vi "BonOMM-SAOMM.vi"() -> ()   [LabVIEW 2019] (continued)
                                n2799 = Two Button Dialog(message="Voulez-vous vraiment utiliser ces \nvaleurs comme valeurs de centre (x,y)", 1:"Non" ("F button name (\"Cancel\")"), 2:"Oui" ("T button name (\"OK\")")) -> (T button?=w6859:bool)
                                n2800 = case shown="Faux" w6859 {
                                tunnel: w6858 -> [w6863 _]
                                tunnel: w6857 -> [w6864 _]
                                frame False {
                                n2801 = local write "Reference Y"(w6864) -> ()
                                n2802 = local write "Reference X"(w6863) -> ()
                                }
                                frame True {
                                }
                                }
                                }
                                }
                                }
                                }
                              }
                            }
                          }
                        }
                      }
                      frame #4 {
                        n2803 = control-ref of="PrAMS-ACK"() -> (w6876:refnum<vi>)
                        n2804 = local read "PrAMS VRN"() -> (w6899:refnum<visa-resource-name>)
                        n2805 = local read "PrAMS Error"() -> (w6898:errorcluster)
                        n2806 = local read "MessageType"() -> (w6884:cluster{string[], u32[]})
                        n2807 = control-ref of="PrAMS actif"() -> (w6877:refnum<vi>)
                        n2808 = local read "Signature"() -> (w6887:u32)
                        n2809 = call-poly "SAOMM-Num2littleEndian.vi"("Number"=w6874) -> ("LiitleEndianedData"=w6883:u8[])  [unwired: 14 in]
                        n2810 = call-poly "SAOMM-Num2littleEndian.vi"("Number"=w6873) -> ("LiitleEndianedData"=w6882:u8[])  [unwired: 14 in]
                        n2811 = call-poly "SAOMM-Num2littleEndian.vi"("Number"=w6868) -> ("LiitleEndianedData"=w6881:u8[])  [unwired: 14 in]
                        n2812 = call-poly "SAOMM-Num2littleEndian.vi"("Number"=w6867) -> ("LiitleEndianedData"=w6880:u8[])  [unwired: 14 in]
                        n2813 = call-poly "SAOMM-Num2littleEndian.vi"("Number"=w6866) -> ("LiitleEndianedData"=w6879:u8[])  [unwired: 14 in]
                        n2814 = call-poly "SAOMM-Num2littleEndian.vi"("Number"=w6865) -> ("LiitleEndianedData"=w6878:u8[])  [unwired: 14 in]
                        n2815 = call "SAOMM-SendSET.vi"("PRAMMS-COMM IN"=w6899, "Active Refnum"=w6877, "PrAMS-ACK"=w6876, "Signature"=w6887, "Error IN"=w6898, "MessageType"=w6884, "Active SET"="emtSetROIHeight", "Value (little endianed byte array)"=w6883) -> ("PRAMMS-COMM OUT"=w6897:refnum<visa-resource-name>, "Error OUT"=w6894:errorcluster)  [unwired: 4 in, 2 out]
                        n2816 = call "SAOMM-SendSET.vi"("PRAMMS-COMM IN"=w6897, "Active Refnum"=w6877, "PrAMS-ACK"=w6876, "Signature"=w6887, "Error IN"=w6894, "MessageType"=w6884, "Active SET"="emtSetROIWidth", "Value (little endianed byte array)"=w6882) -> ("PRAMMS-COMM OUT"=w6896:refnum<visa-resource-name>, "Error OUT"=w6893:errorcluster)  [unwired: 4 in, 2 out]
                        n2817 = call "SAOMM-SendSET.vi"("PRAMMS-COMM IN"=w6896, "Active Refnum"=w6877, "PrAMS-ACK"=w6876, "Signature"=w6887, "Error IN"=w6893, "MessageType"=w6884, "Active SET"="emtSetROIXReferencePoint", "Value (little endianed byte array)"=w6881) -> ("PRAMMS-COMM OUT"=w6895:refnum<visa-resource-name>, "Error OUT"=w6892:errorcluster)  [unwired: 4 in, 2 out]
                        n2818 = call "SAOMM-SendSET.vi"("PRAMMS-COMM IN"=w6895, "Active Refnum"=w6877, "PrAMS-ACK"=w6876, "Signature"=w6887, "Error IN"=w6892, "MessageType"=w6884, "Active SET"="emtSetROIYReferencePoint", "Value (little endianed byte array)"=w6880) -> ("PRAMMS-COMM OUT"=w6889:refnum<visa-resource-name>, "Error OUT"=w6888:errorcluster)  [unwired: 4 in, 2 out]
                        n2819 = call "SAOMM-SendSET.vi"("PRAMMS-COMM IN"=w6889, "Active Refnum"=w6877, "PrAMS-ACK"=w6876, "Signature"=w6887, "Error IN"=w6888, "MessageType"=w6884, "Active SET"="emtSetROIXOffset", "Value (little endianed byte array)"=w6879) -> ("PRAMMS-COMM OUT"=w6890:refnum<visa-resource-name>, "Error OUT"=w6891:errorcluster)  [unwired: 4 in, 2 out]
                        n2820 = call "SAOMM-SendSET.vi"("PRAMMS-COMM IN"=w6890, "Active Refnum"=w6877, "PrAMS-ACK"=w6876, "Signature"=w6887, "Error IN"=w6891, "MessageType"=w6884, "Active SET"="emtSetROIYOffset", "Value (little endianed byte array)"=w6878) -> ("Error OUT"=w6875:errorcluster)  [unwired: 4 in, 3 out]
                        n2821 = local write "PrAMS Error"(w6875) -> ()
                      }
                      frame #5 {
                        # "Pas certain que ce soit encore très utile ..."
                        n2822 = local write "Centrage_ready"(TRUE) -> ()
                        n2823 = global write "Globals.vi" "EXIT"(FALSE) -> ()
                        n2824 = local write "Indicateur d'état"("Centrage : fin de la routine" ("Indicateur d'état")) -> ()
                      }
                    }
                  }
                }
                n2825 = flat-sequence {
                  tunnel: [FALSE ("CentrageLed")] -> w6632
                  frame #0 {
                    "Centrage_ready" <- FALSE
                  }
                  frame #1 {
                    n2826 = while {
                      stop <- w6905 stop-if-true
                      n2827 = local read "CentrageLed"() -> (w6907:bool)
                      n2828 = Wait (ms)(milliseconds to wait=u32 250) -> ()  [unwired: 1 out]
                      n2829 = Not(x=w6907) -> (.not. x?=→"CentrageLed":bool)
                      n2830 = local read "Centrage_ready"() -> (w6905:bool)
                    }
                  }
                }
                n2831 = global write "Globals.vi" "EXIT"(FALSE ("Visible")) -> ()
                n2832 = local write "CentrageLed"(w6632) -> ()
              }
              event "ST+", "ST-": Value Change {
                n2833 = event-data() -> ()  [unwired: 1 in, 6 out]
                n2834 = Build Array("ST+", "ST-") -> (w6911:bool[])
                n2835 = Boolean Array To Number(Boolean array=w6911) -> (number=w6910:u32)
                n2836 = local read "MC-BonOMM VRN"() -> (w6909:refnum<visa-resource-name>)
                n2837 = case shown="2" w6910 {
                  tunnel: w6909 -> [_ w6916 w6936]
                  frame 0, Default {
                  }
                  frame 2 {
                    n2838 = call "MC-BonOMM_talker.vi"("MC-BonOMM VRN"=w6916, "Commande"="-" ("write buffer"), "Timeout (ms)"=1000, "answer=command?"=TRUE) -> ("ok ?"=w6914:bool)  [unwired: 1 in, 1 out]
                    n2839 = case shown="Vrai" w6914 {
                      tunnel: w6916 -> [w6919 w6930]
                      frame False {
                        n2840 = One Button Dialog(message="Erreur lors de la commande de déplacement", button name ("OK")="Ok ?!?") -> ()  [unwired: 1 out]
                        n2841 = call "MC-BonOMM_talker.vi"("MC-BonOMM VRN"=w6919, "Commande"="s" ("write buffer"), "Timeout (ms)"=1000, "answer=command?"=TRUE) -> ()  [unwired: 1 in, 2 out]
                      }
                      frame True {
                        n2842 = while {
                          tunnel: w6930 -> [w6932]
                          tunnel: [w6932] -> w6929
                          stop <- w6931 continue-if-true
                          n2843 = local read "ST-"() -> (w6931:bool)
                          n2844 = Wait (ms)(milliseconds to wait=u32 50) -> ()  [unwired: 1 out]
                        }
                        n2845 = call "MC-BonOMM_talker.vi"("MC-BonOMM VRN"=w6929, "Commande"="s" ("write buffer"), "Timeout (ms)"=1000, "answer=command?"=TRUE) -> ("ok ?"=w6925:bool)  [unwired: 1 in, 1 out]
                        n2846 = local write "MC_connect"(w6925) -> ()
                      }
                    }
                    n2847 = local write "MC_connect"(w6914) -> ()
                  }
                  frame 1 {
                    n2848 = call "MC-BonOMM_talker.vi"("MC-BonOMM VRN"=w6936, "Commande"="+" ("write buffer"), "Timeout (ms)"=1000, "answer=command?"=TRUE) -> ("ok ?"=w6934:bool)  [unwired: 1 in, 1 out]
                    n2849 = case shown="Vrai" w6934 {
                      tunnel: w6936 -> [w6940 w6951]
                      frame False {
                        n2850 = One Button Dialog(message="Erreur lors de la commande de déplacement", button name ("OK")="Ok ?!?") -> ()  [unwired: 1 out]
                        n2851 = call "MC-BonOMM_talker.vi"("MC-BonOMM VRN"=w6940, "Commande"="s" ("write buffer"), "Timeout (ms)"=1000, "answer=command?"=TRUE) -> ("ok ?"=w6939:bool)  [unwired: 1 in, 1 out]
                        n2852 = local write "MC_connect"(w6939) -> ()
                      }
                      frame True {
                        n2853 = while {
                          tunnel: w6951 -> [w6953]
                          tunnel: [w6953] -> w6950
                          stop <- w6952 continue-if-true
                          n2854 = local read "ST+"() -> (w6952:bool)
                          n2855 = Wait (ms)(milliseconds to wait=u32 50) -> ()  [unwired: 1 out]
                        }
                        n2856 = call "MC-BonOMM_talker.vi"("MC-BonOMM VRN"=w6950, "Commande"="s" ("write buffer"), "Timeout (ms)"=1000, "answer=command?"=TRUE) -> ("ok ?"=w6946:bool)  [unwired: 1 in, 1 out]
                        n2857 = local write "MC_connect"(w6946) -> ()
                      }
                    }
                    n2858 = local write "MC_connect"(w6934) -> ()
                  }
                }
              }
              event "Ajust z to tel": Value Change {
                n2859 = event-data() -> ()  [unwired: 1 in, 6 out]
                n2860 = local read "Foyer"() -> (w6955:dbl)
                n2861 = case shown="Vrai" "Ajust z to tel" {
                  tunnel: w6955 -> [_ w6971]
                  frame False {
                  }
                  frame True {
                    n2862 = local read "k0_focus"() -> (w6967:dbl)
                    n2863 = local read "k1_focus"() -> (w6966:dbl)
                    n2864 = formula code="foyersonde=foyertel*k1+k0;"("foyertel"=w6971, "k0"=w6967, "k1"=w6966) -> ("foyersonde"=w6958:dbl)
                    n2865 = local read "CentreTel X"() -> (w6965:dbl)
                    n2866 = local read "CentreTel Y"() -> (w6964:dbl)
                    n2867 = local read "Position X"() -> (w6960:dbl)
                    n2868 = local read "Position Y"() -> (w6959:dbl)
                    n2869 = local read "a1_focus"() -> (w6963:dbl)
                    n2870 = local read "a2_focus"() -> (w6962:dbl)
                    n2871 = local read "a3_focus"() -> (w6961:dbl)
                    n2872 = control-ref of="TERMINAL"() -> (w6969:refnum<vi>)
                    n2873 = control-ref of="Indicateur d'état"() -> (w6970:refnum<vi>)
                    n2874 = call "Calc_focus.vi"("Pos X"=w6960, "a0"=w6958, "Pos Y"=w6959, "Cen X"=w6965, "Cen Y"=w6964, "a1"=w6963, "a2"=w6962, "a3"=w6961) -> ("Foyer"=w6957:dbl)  [unwired: 6 in, 1 out]
                    n2875 = call "TERMINAL.vi"("Indicateur Refnum"=w6970, "Terminal Refnum"=w6969, "Indicateur d'état"="Ajustement automatique du foyer de la caméra de guidage") -> ()
                    n2876 = local write "FoyerAuCentre"(w6958) -> ()
                    n2877 = property on="FoyerTable" class="NumNb (strict)"("Val(Sgnl)"=w6957) -> ()  [unwired: 2 in, 2 out]
                  }
                }
              }
              event "Foyer+", "Foyer-": Mouse Down {
                n2878 = event-data() -> ()  [unwired: 1 in, 8 out]
                n2879 = Or(x="Foyer+", y="Foyer-") -> (x .or. y?=w6973:bool)
                n2880 = case shown="Vrai" w6973 {
                  tunnel: "Foyer+" -> [_ w6997]
                  frame False {
                  }
                  frame True {
                    w6983 = "AZ" ("StageTag")
                    n2881 = local read "vitesse focus"() -> (w6996:dbl)
                    n2882 = control-ref of="TERMINAL"() -> (w6988:refnum<vi>)
                    n2883 = control-ref of="Indicateur d'état"() -> (w6987:refnum<vi>)
                    n2884 = Negate(x=w6996) -> (-x=w6995:dbl)
                    n2885 = local write "Focusing"(TRUE ("Focusing")) -> ()
                    n2886 = Select(t=w6996, s=w6997, f=w6995) -> (s? t:f=w6982:dbl)
                    n2887 = local read "Table VRN"() -> (w6994:refnum<visa-resource-name>)
                    n2888 = local read "Table Error"() -> (w6993:errorcluster)
                    n2889 = call "TERMINAL.vi"("Indicateur Refnum"=w6987, "Terminal Refnum"=w6988, "Indicateur d'état"="Modification du foyer \"au centre\" de la caméra de guidage") -> ()
                    n2890 = control-ref of="Table actif"() -> (w6990:refnum<vi>)
                    n2891 = call "Newmark-Jog.vi"("Table VRN IN"=w6994, "StageTag"=w6983, "Bool Refnum"=w6990, "Error IN"=w6993, "Velocity"=w6982) -> ("Table VRN OUT"=w6991:refnum<visa-resource-name>, "Error OUT"=w6992:errorcluster)  [unwired: 9 in]
                    n2892 = flat-sequence {
                      tunnel: w6991 -> [w7001]
                      tunnel: w6992 -> [w7000]
                      tunnel: [w7001] -> w6986
                      tunnel: [w7000] -> w6985
                      tunnel: [w6999] -> w6984
                      tunnel: w6983 -> [w6999]
                      tunnel: [w6998] -> _
                      tunnel: w6985 -> [w7013]
                      tunnel: w6986 -> [w7014]
                      tunnel: [w7011] -> w6981
                      tunnel: [w7010] -> w6979
                      tunnel: [w7012] -> w6977
                      tunnel: w6984 -> [w7012]
                      tunnel: w6981 -> [w7018]
                      tunnel: [w7018] -> w6980
                      tunnel: w6979 -> [w7017]
                      tunnel: [w7017] -> w6978
                      tunnel: w6977 -> [w7016]
                      tunnel: [w7016] -> w6976
                      tunnel: w6980 -> [w7029]
                      tunnel: w6978 -> [w7028]
                      tunnel: w6976 -> [w7027]
                      frame #0 {
                        n2893 = while {
                          tunnel: [w7002] -> w6998
                          stop <- w7004 continue-if-true
                          n2894 = local read "Exceptions"() -> (w7003:T3)
                          n2895 = local read "Foyer-"() -> (w7007:bool)
                          n2896 = local read "Foyer+"() -> (w7008:bool)
                          n2897 = Unbundle By Name(w7003) -> ("Overtravel"=w7002:bool)
                          n2898 = Or(x=w7008, y=w7007) -> (x .or. y?=w7005:bool)
                          n2899 = Wait (ms)(milliseconds to wait=u32 100) -> ()  [unwired: 1 out]
                          n2900 = Not(x=w7002) -> (.not. x?=w7006:bool)
                          n2901 = And(x=w7005, y=w7006) -> (x .and. y?=w7004:bool)
                        }
                      }
                      frame #1 {
                        n2902 = control-ref of="Table actif"() -> (w7015:refnum<vi>)
                        n2903 = call "Newmark-Stop.vi"("Table VRN IN"=w7014, "Bool Refnum"=w7015, "Error IN"=w7013) -> ("Table VRN OUT"=w7011:refnum<visa-resource-name>, "Error OUT"=w7010:errorcluster)  [unwired: 11 in]
                      }
                      frame #2 {
                        n2904 = while {
                          stop <- w7020 continue-if-true
                          n2905 = local read "MovingZ"() -> (w7020:bool)
                          n2906 = Wait (ms)(milliseconds to wait=u32 100) -> ()  [unwired: 1 out]
                        }
                      }
                      frame #3 {
                        n2907 = local read "vitesse rapide"() -> (w7024:dbl)
                        n2908 = local read "vitesse lente"() -> (w7025:dbl)
                        n2909 = local read "accelleration"() -> (w7023:dbl)
                        n2910 = control-ref of="Table actif"() -> (w7026:refnum<vi>)
                        n2911 = call "Newmark-SetSpeed.vi"("Table VRN"=w7029, "StageTAG"=w7027, "Bool Refnum"=w7026, "Error IN"=w7028, "Vitesse Lente"=w7025, "Vitesse Rapide"=w7024, "Accélération"=w7023) -> ("Table VRN OUT"=w7022:refnum<visa-resource-name>, "Error OUT"=w7021:errorcluster)  [unwired: 6 in, 1 out]
                        n2912 = local write "Table VRN"(w7022) -> ()
                        n2913 = local write "Table Error"(w7021) -> ()
                      }
                    }
                  }
                }
              }
              event "FoyerTable": Value Change {
                n2914 = event-data() -> ("NewVal"=w7032:dbl)  [unwired: 1 in, 5 out]
                n2915 = local write "Cible Z"(w7032) -> ()
                n2916 = local read "Table VRN"() -> (w7039:refnum<visa-resource-name>)
                n2917 = local read "Table Error"() -> (w7037:errorcluster)
                n2918 = control-ref of="Table actif"() -> (w7035:refnum<vi>)
                n2919 = local write "CorrectZ"(TRUE ("CorrectZ")) -> ()
                n2920 = call "Newmark-GotoOne.vi"("Table VRN IN"=w7039, "Bool Refnum"=w7035, "StageTAG"="AZ", "Notify?"=FALSE, "Error IN"=w7037, "Position"=w7032) -> ("Table VRN OUT"=w7038:refnum<visa-resource-name>, "Error OUT"=w7036:errorcluster)  [unwired: 8 in]
                n2921 = local write "Focusing"(TRUE ("Focusing")) -> ()
                n2922 = local write "Table VRN"(w7038) -> ()
                n2923 = local write "Table Error"(w7036) -> ()
                n2924 = Unbundle By Name(w7036) -> ("status"=w7040:bool)
                n2925 = Not(x=w7040) -> ()  [unwired: 1 out]
              }
              event "ApplyCorrection": Value Change {
                n2926 = event-data() -> ()  [unwired: 1 in, 6 out]
                n2927 = local read "ApplyCorrection"() -> (w7041:bool)
                n2928 = case shown="Vrai" w7041 {
                  frame False {
                  }
                  frame True {
                    n2929 = local read "Cible X"() -> (w7047:dbl)
                    n2930 = local read "Position X"() -> (w7044:dbl)
                    n2931 = local read "Cible Y"() -> (w7045:dbl)
                    n2932 = local read "Position Y"() -> (w7046:dbl)
                    n2933 = local read "Cible Z"() -> (w7049:dbl)
                    n2934 = local read "Position Z"() -> (w7048:dbl)
                    n2935 = Subtract(x=w7045, y=w7046) -> (x-y=w7042:dbl)
                    n2936 = Subtract(x=w7047, y=w7044) -> (x-y=w7043:dbl)
                    n2937 = Subtract(x=w7049, y=w7048) -> (x-y=w7053:dbl)
                    n2938 = local read "Table Error"() -> (w7057:errorcluster)
                    n2939 = local read "Table VRN"() -> (w7058:refnum<visa-resource-name>)
                    n2940 = Build Array(w7043, w7042, w7053) -> (w7052:dbl[])
                    n2941 = control-ref of="Table actif"() -> (w7056:refnum<vi>)
                    n2942 = local write "ApplyCorrection"(FALSE ("Correct")) -> ()
                    n2943 = call "Newmark-CorrectPosition.vi"("Table VRN IN"=w7058, "Bool Refnum"=w7056, "Error IN"=w7057, "StageTags"=string[] ["AX", "AY", "AZ"], "Corrections"=w7052) -> ("Table VRN OUT"=w7055:refnum<visa-resource-name>, "Error OUT"=w7054:errorcluster)  [unwired: 8 in, 1 out]
                    n2944 = local write "Table VRN"(w7055) -> ()
                    n2945 = local write "Table Error"(w7054) -> ()
                  }
                }
              }
              event "YReference", "XReference": Value Change {
                n2946 = event-data() -> ()  [unwired: 1 in, 6 out]
                n2947 = control-ref of="ImgArray"() -> (w7067:refnum<vi>)
                n2948 = local read "ROIHeight"() -> (w7065:u16)
                n2949 = local read "ROIWidth"() -> (w7066:u16)
                n2950 = call "SAOMM-Cursor2ROI.vi"("ImgRef"=w7067, "CursorX"="XReference", "CursorY"="YReference", "ROIWidth"=w7066, "ROIHeight"=w7065) -> ("ROIXOffset"=w7064:u16, "ROIYOffset"=w7063:u16)  [unwired: 7 in, 2 out]
                n2951 = flat-sequence {
                  tunnel: w7064 -> [w7069]
                  tunnel: w7063 -> [w7068]
                  tunnel: [w7069] -> w7060
                  tunnel: [w7068] -> w7059
                  tunnel: w7060 -> [w7075]
                  tunnel: w7059 -> [w7074]
                  frame #0 {
                    n2952 = local write "ROIXOffset"(w7069) -> ()
                    n2953 = local write "ROIYOffset"(w7068) -> ()
                  }
                  frame #1 {
                    n2954 = local read "Binning"() -> (w7095:u16)
                    n2955 = local read "ROIWidth"() -> (w7089:u16)
                    n2956 = local read "ROIHeight"() -> (w7090:u16)
                    n2957 = local read "Naxis1"() -> (w7093:u16)
                    n2958 = local read "Naxis2"() -> (w7092:u16)
                    n2959 = local read "XROIRef"() -> (w7087:dbl)
                    n2960 = local read "YROIRef"() -> (w7073:dbl)
                    n2961 = Bundle("ROIXOffset"=w7075, "ROIYOffset"=w7074) -> (w7091:cluster{"ROIXOffset":u16, "ROIYOffset":u16})  [unwired: 1 in]
                    n2962 = Bundle("Naxis1"=w7093, "Naxis2"=w7092) -> (w7094:cluster{"Naxis1":u16, "Naxis2":u16})  [unwired: 1 in]
                    n2963 = Bundle("ROIWidth"=w7089, "ROIHeight"=w7090) -> (w7070:cluster{"ROIWidth":u16, "ROIHeight":u16})  [unwired: 1 in]
                    n2964 = Bundle("XROIRef"=w7087, "YROIRef"=w7073) -> (w7088:cluster{"XROIRef":dbl, "YROIRef":dbl})  [unwired: 1 in]
                    n2965 = call "SAOMM-ROI_Fixer.vi"("Binning"=w7095, "Use Offset?"=TRUE, "naxis"=w7094, "ROI"=w7070, "Offset"=w7091, "Reference Pixel"=w7088) -> ("FixedOffset"=w7078:cluster{"ROIXOffset":u16, "ROIYOffset":u16}, "FixedPixel"=w7076:cluster{"PixelX":dbl, "PixelY":dbl})  [unwired: 6 in, 2 out]
                    n2966 = Unbundle By Name(w7078) -> ("ROIXOffset"=w7086:u16, "ROIYOffset"=w7085:u16)
                    n2967 = control-ref of="PrAMS-ACK"() -> (w7098:refnum<vi>)
                    n2968 = local read "MessageType"() -> (w7097:cluster{string[], u32[]})
                    n2969 = control-ref of="PrAMS actif"() -> (w7103:refnum<vi>)
                    n2970 = local read "PrAMS VRN"() -> (w7102:refnum<visa-resource-name>)
                    n2971 = local read "PrAMS Error"() -> (w7101:errorcluster)
                    n2972 = Unbundle By Name(w7076) -> ("PixelX"=w7079:dbl, "PixelY"=w7082:dbl)
                    n2973 = To Double Precision Float(number=w7086) -> (double precision float=w7081:dbl)
                    n2974 = To Double Precision Float(number=w7085) -> (double precision float=w7080:dbl)
                    n2975 = Bundle("ROIYOffset"=w7085, "ROIXOffset"=w7086) -> (w7077:cluster{"ROIYOffset":u16, "ROIXOffset":u16})  [unwired: 1 in]
                    n2976 = Add(x=w7080, y=w7079) -> (x+y=w7072:dbl)
                    n2977 = Add(x=w7081, y=w7082) -> (x+y=w7071:dbl)
                    n2978 = call "SAOMM-UpdateROI.vi"("PRAMMS-COMM IN"=w7102, "Active Refnum"=w7103, "PrAMS-ACK"=w7098, "MessageType"=w7097, "Error IN"=w7101, "Position"=w7077) -> ("PRAMMS-COMM OUT"=w7100:refnum<visa-resource-name>, "Error OUT"=w7099:errorcluster)  [unwired: 7 in, 1 out]
                    n2979 = property on="ImgArray" class="GraphInt (strict)"() -> ("Cursor.Cursor Position"=w7084:T45)  [unwired: 2 in, 2 out]
                    n2980 = local write "XReference"(w7072) -> ()
                    n2981 = local write "YReference"(w7071) -> ()
                    n2982 = local write "PrAMS Error"(w7099) -> ()
                    n2983 = local write "PrAMS VRN"(w7100) -> ()
                    n2984 = Bundle(cluster=w7084, "Cursor X"=w7072, "Cursor Y"=w7071) -> (w7083:T45)
                    n2985 = property on="ImgArray" class="GraphInt (strict)"("Cursor.Cursor Position"=w7083) -> ()  [unwired: 2 in, 2 out]
                  }
                }
              }
              event "go Ouest", "go Nord", "go Est", "go Sud": Mouse Down {
                n2986 = event-data() -> ()  [unwired: 1 in, 8 out]
                n2987 = Compound Arithmetic op=OR("go Nord", "go Sud", "go Est", "go Ouest") -> (w7104:bool)
                n2988 = local write "enfoncé"(w7104) -> ()
                n2989 = case shown="Vrai" w7104 {
                  tunnel: "go Nord" -> [_ w7113]
                  tunnel: "go Sud" -> [_ w7112]
                  tunnel: "go Est" -> [_ w7111]
                  tunnel: "go Ouest" -> [_ w7110]
                  frame False {
                  }
                  frame True {
                    n2990 = local read "act_sonde"() -> (w7109:bool)
                    n2991 = Build Array(w7113, w7112, w7111, w7110) -> (w7115:bool[])
                    n2992 = Boolean Array To Number(Boolean array=w7115) -> (number=w7114:u32)
                    n2993 = case shown="Vrai" w7109 {
                      tunnel: w7114 -> [w7121 w7178]
                      frame False {
                        # "0.1=1'/sec"
                        n2994 = local read "FieldAstrom"() -> (w7119:T4)
                        n2995 = local read "ImgAstrom"() -> (w7118:T4)
                        n2996 = while {
                          tunnel: w7121 -> [w7139]
                          tunnel: 0.1 ("t") -> [w7136]
                          tunnel: w7119 -> [w7130]
                          tunnel: w7118 -> [w7133]
                          tunnel: [FALSE] -> w7117
                          tunnel: u32 0 ("Active Cursor") -> [w7122]
                          stop <- w7134 continue-if-true
                          n2997 = property on="TableXYPos" class="GraphXY (strict)"("Active Cursor"=w7122) -> (error out=w7126:errorcluster)  [unwired: 2 in, 1 out]
                          n2998 = property on="TableXYPos" class="GraphXY (strict)"(error in=w7126) -> (error out=w7124:errorcluster, "Cursor.Cursor Position"=w7125:T45)  [unwired: 1 in, 1 out]
                          n2999 = Unbundle(w7125) -> ("Cursor X"=w7138:dbl, "Cursor Y"=w7137:dbl)
                          n3000 = case shown="0, Par défaut" w7139 {
                            tunnel: [w7161 w7162 w7166 w7171 w7175] -> w7131
                            tunnel: w7138 -> [w7161 w7162 w7166 w7173 w7177]
                            tunnel: [w7160 w7163 w7168 w7170 w7176] -> w7132
                            tunnel: w7137 -> [w7160 w7165 w7167 w7170 w7176]
                            tunnel: w7136 -> [_ w7164 w7169 w7172 w7174]
                            frame 0, Default {
                            }
                            frame 1 {
                              n3001 = Add(x=w7165, y=w7164) -> (x+y=w7163:dbl)
                            }
                            frame 2 {
                              n3002 = Subtract(x=w7167, y=w7169) -> (x-y=w7168:dbl)
                            }
                            frame 4 {
                              n3003 = Add(x=w7173, y=w7172) -> (x+y=w7171:dbl)
                            }
                            frame 8 {
                              n3004 = Subtract(x=w7177, y=w7174) -> (x-y=w7175:dbl)
                            }
                          }
                          n3005 = Wait (ms)(milliseconds to wait=u32 100) -> ()  [unwired: 1 out]
                          n3006 = Bundle("Cursor X"=w7131, "Cursor Y"=w7132) -> (w7140:cluster{"Cursor X":dbl, "Cursor Y":dbl})  [unwired: 1 in]
                          n3007 = property on="TableXYPos" class="GraphXY (strict)"(error in=w7124, "Cursor.Cursor Position"=w7140) -> ()  [unwired: 1 in, 2 out]
                          n3008 = call "xy2ad.vi"("Y (px)"=w7132, "X (px)"=w7131, "Astrometry"=w7130) -> ("DEC (°)"=w7128:dbl, "RA (°)"=w7129:dbl)  [unwired: 5 in, 2 out]
                          n3009 = local read "ImageDSSLed"() -> (w7123:bool)
                          n3010 = case shown="Vrai" w7123 {
                            tunnel: w7133 -> [_ w7149]
                            tunnel: w7129 -> [_ w7148]
                            tunnel: w7128 -> [_ w7147]
                            frame False {
                            }
                            frame True {
                              w7145 = u16 1 items=["Region d'intérêt", "Prévisualisation", "Idle"] ("ImageUsage")
                              n3011 = call "ad2xy.vi"("DEC"=w7147, "RA"=w7148, "Astrometry"=w7149) -> ("Y"=w7151:dbl, "X"=w7152:dbl)  [unwired: 6 in, 1 out]
                              n3012 = local read "ImgData"() -> (w7157:sgl[][])
                              n3013 = To Long Integer(number=w7152) -> (32bit integer=w7155:i32)
                              n3014 = To Long Integer(number=w7151) -> (32bit integer=w7156:i32)
                              n3015 = call "subimage.vi"("Ysz/2"=100 ("Xsz/2"), "Xsz/2"=100, "Yc"=w7156, "Xc"=w7155, "ImgData"=w7157) -> ("SubImg"=w7158:sgl[][])  [unwired: 6 in]
                              n3016 = local write "SubIMG4DSS?"(TRUE ("SubIMG4DSS?")) -> ()
                              n3017 = Array Max & Min(array=w7158) -> (max value=w7159:sgl)  [unwired: 3 out]
                              n3018 = local write "ImageUsage"(w7145) -> ()
                              n3019 = call "Draw_crosshair.vi"("Image IN"=w7158, "White Value"=w7159) -> ("Image OUT"=w7150:sgl[][])  [unwired: 13 in]
                              n3020 = local write "subimg"(w7150) -> ()
                            }
                          }
                          n3021 = local read "go Nord"() -> (w7142:bool)
                          n3022 = local read "go Ouest"() -> (w7144:bool)
                          n3023 = local read "go Est"() -> (w7143:bool)
                          n3024 = local read "go Sud"() -> (w7141:bool)
                          n3025 = Compound Arithmetic op=OR(w7144, w7143, w7142, w7141) -> (w7134:bool)
                          n3026 = local write "enfoncé"(w7134) -> ()
                        }
                        n3027 = local write "go Nord"(w7117) -> ()
                        n3028 = local write "go Ouest"(w7117) -> ()
                        n3029 = local write "go Est"(w7117) -> ()
                        n3030 = local write "go Sud"(w7117) -> ()
                        n3031 = local write "enfoncé"(w7117) -> ()
                      }
                      frame True {
                        n3032 = flat-sequence {
                          tunnel: w7178 -> [w7180]
                          frame #0 {
                            # "Vrai = buggy continuous\nFaux = nouveau pas-à-pas"
                            n3033 = case shown="Faux" FALSE {
                              tunnel: w7180 -> [w7182 w7227]
                              frame False {
                                n3034 = flat-sequence {
                                tunnel: w7182 -> [w7184]
                                tunnel: [w7184] -> w7181
                                tunnel: w7181 -> [w7203]
                                frame #0 {
                                w7183 = FALSE ("go Ouest")
                                n3035 = local write "go Nord"(w7183) -> ()
                                n3036 = local write "go Ouest"(w7183) -> ()
                                n3037 = local write "go Est"(w7183) -> ()
                                n3038 = local write "go Sud"(w7183) -> ()
                                n3039 = local write "enfoncé"(w7183) -> ()
                                }
                                frame #1 {
                                # "Devrait être remplacé par la valeur théorique ..."
                                n3040 = property on="TableXYPos" class="GraphXY (strict)"("Active Cursor"=u32 1) -> (error out=w7206:errorcluster)  [unwired: 2 in, 1 out]
                                n3041 = property on="TableXYPos" class="GraphXY (strict)"(error in=w7206) -> ("Cursor.Cursor Position"=w7204:T45)  [unwired: 1 in, 2 out]
                                n3042 = Unbundle(w7204) -> ("Cursor X"=w7208:dbl, "Cursor Y"=w7207:dbl)
                                n3043 = case shown="1" w7203 {
                                tunnel: [w7210 w7211 w7215 w7220 w7224] -> w7201
                                tunnel: w7208 -> [w7210 w7211 w7215 w7222 w7226]
                                tunnel: [w7209 w7212 w7217 w7219 w7225] -> w7200
                                tunnel: w7207 -> [w7209 w7214 w7216 w7219 w7225]
                                tunnel: "ClickJOG" -> [_ w7213 w7218 w7221 w7223]
                                frame 0, Default {
                                }
                                frame 1 {
                                n3044 = Add(x=w7214, y=w7213) -> (x+y=w7212:dbl)
                                }
                                frame 2 {
                                n3045 = Subtract(x=w7216, y=w7218) -> (x-y=w7217:dbl)
                                }
                                frame 4 {
                                n3046 = Add(x=w7222, y=w7221) -> (x+y=w7220:dbl)
                                }
                                frame 8 {
                                n3047 = Subtract(x=w7226, y=w7223) -> (x-y=w7224:dbl)
                                }
                                }
                                n3048 = local read "BrasPesto"() -> (w7186:bool)
                                n3049 = local read "LimXPesto"() -> (w7185:dbl)
                                n3050 = local read "FieldAstrom"() -> (w7199:T4)
                                n3051 = call "xy2ad.vi"("Y (px)"=w7200, "X (px)"=w7201, "Astrometry"=w7199) -> ("DEC (°)"=w7197:dbl, "RA (°)"=w7198:dbl)  [unwired: 5 in, 2 out]
                                n3052 = local read "Position Z"() -> (w7193:dbl)
                                n3053 = local read "TableAstrom"() -> (w7196:T4)
                                n3054 = call "ad2xy.vi"("DEC"=w7197, "RA"=w7198, "Astrometry"=w7196) -> ("Y"=w7195:dbl, "X"=w7194:dbl)  [unwired: 6 in, 1 out]
                                n3055 = local read "Table VRN"() -> (w7191:refnum<visa-resource-name>)
                                n3056 = local read "Table Error"() -> (w7190:errorcluster)
                                n3057 = control-ref of="Table actif"() -> (w7192:refnum<vi>)
                                n3058 = call "Newmark-GotoAll.vi"("Table VRN IN"=w7191, "BrasPesto"=w7186, "Bool Refnum"=w7192, "LimXPesto"=w7185, "Notify?"=FALSE, "Error IN"=w7190, "Position X"=w7194, "Position Y"=w7195, "Position Z"=w7193) -> ("Table VRN OUT"=w7189:refnum<visa-resource-name>, "Error OUT"=w7188:errorcluster)  [unwired: 5 in]
                                n3059 = local write "Table Error"(w7188) -> ()
                                n3060 = local write "Table VRN"(w7189) -> ()
                                n3061 = local write "Cible X"(w7194) -> ()
                                n3062 = local write "Cible Z"(w7193) -> ()
                                n3063 = local write "Cible Y"(w7195) -> ()
                                }
                                }
                              }
                              frame True {
                                n3064 = stacked-sequence {
                                tunnel: w7227 -> [w7241 _]
                                frame #0 {
                                # "Est (180)"
                                # "Ouest (0)"
                                # "Sud (270)"
                                # "Nord (90)"
                                n3065 = case shown="2" w7241 {
                                tunnel: [45.0 90.0 270.0 180.0 0.0] -> w7240
                                frame Default {
                                }
                                frame 1 {
                                # "Nord"
                                }
                                frame 2 {
                                # "Sud"
                                }
                                frame 4 {
                                # "Est"
                                }
                                frame 8 {
                                # "Ouest"
                                }
                                }
                                n3066 = local read "RotationEffective"() -> (w7242:dbl)
                                n3067 = local read "Position X"() -> (w7239:dbl)
                                n3068 = local read "Position Y"() -> (w7238:dbl)
                                n3069 = call "FieldInterference.vi"("XCorner"=dbl[] [0.0, 500000.0, 500000.0, 0.0], "Rotation"=w7242, "YCorner"=dbl[] [0.0, 0.0, 500000.0, 500000.0], "Xsonde"=w7239, "Ysonde"=w7238, "Direction"=w7240) -> ("XCible"=w7235:dbl, "YCible"=w7234:dbl)  [unwired: 6 in, 2 out]
                                n3070 = local read "vitesse jog"() -> (w7228:dbl)
                                n3071 = local read "Table VRN"() -> (w7230:refnum<visa-resource-name>)
                                n3072 = control-ref of="Table actif"() -> (w7229:refnum<vi>)
                                n3073 = local read "Table Error"() -> (w7231:errorcluster)
                                n3074 = call "Newmark-JogLinear.vi"("Table VRN IN"=w7230, "Bool Refnum"=w7229, "Error IN"=w7231, "Position X"=w7235, "Position Y"=w7234, "Vitesse Jog"=w7228) -> ("Table VRN OUT"=w7233:refnum<visa-resource-name>, "Error OUT"=w7232:errorcluster)  [unwired: 8 in]
                                n3075 = local write "Cible X"(w7235) -> ()
                                n3076 = local write "Table VRN"(w7233) -> ()
                                n3077 = local write "Table Error"(w7232) -> ()
                                n3078 = local write "Cible Y"(w7234) -> ()
                                }
                                frame #1 {
                                n3079 = flat-sequence {
                                frame #0 {
                                n3080 = while {
                                stop <- w7255 continue-if-true
                                n3081 = local read "Exceptions"() -> (w7249:T3)
                                n3082 = local read "go Nord"() -> (w7252:bool)
                                n3083 = local read "go Ouest"() -> (w7254:bool)
                                n3084 = local read "go Est"() -> (w7253:bool)
                                n3085 = local read "go Sud"() -> (w7251:bool)
                                n3086 = Compound Arithmetic op=OR(w7254, w7253, w7252, w7251) -> (w7250:bool)
                                n3087 = Unbundle By Name(w7249) -> ("Overtravel"=w7248:bool)
                                n3088 = Not(x=w7248) -> (.not. x?=w7256:bool)
                                n3089 = Wait (ms)(milliseconds to wait=u32 50) -> ()  [unwired: 1 out]
                                n3090 = And(x=w7250, y=w7256) -> (x .and. y?=w7255:bool)
                                }
                                }
                                frame #1 {
                                n3091 = local read "Table VRN"() -> (w7268:refnum<visa-resource-name>)
                                n3092 = local read "Table Error"() -> (w7267:errorcluster)
                                n3093 = control-ref of="Table actif"() -> (w7258:refnum<vi>)
                                n3094 = local read "vitesse rapide"() -> (w7260:dbl)
                                n3095 = local read "vitesse lente"() -> (w7261:dbl)
                                n3096 = local read "accelleration"() -> (w7259:dbl)
                                n3097 = control-ref of="Table actif"() -> (w7269:refnum<vi>)
                                n3098 = call "Newmark-Stop.vi"("Table VRN IN"=w7268, "Bool Refnum"=w7269, "Error IN"=w7267) -> ("Table VRN OUT"=w7266:refnum<visa-resource-name>, "Error OUT"=w7265:errorcluster)  [unwired: 11 in]
                                n3099 = for {
                                tunnel: w7266 -> [w7278]
                                tunnel: w7265 -> [w7277]
                                tunnel: [w7276] -> w7264
                                tunnel: [w7275] -> w7263
                                tunnel: string[] ["AX", "AY"] -> [w7274] mode=indexing
                                tunnel: w7261 -> [w7273]
                                tunnel: w7260 -> [w7272]
                                tunnel: w7259 -> [w7271]
                                tunnel: w7258 -> [w7270]
                                n3100 = call "Newmark-SetSpeed.vi"("Table VRN"=w7278, "StageTAG"=w7274, "Bool Refnum"=w7270, "Error IN"=w7277, "Vitesse Lente"=w7273, "Vitesse Rapide"=w7272, "Accélération"=w7271) -> ("Table VRN OUT"=w7276:refnum<visa-resource-name>, "Error OUT"=w7275:errorcluster)  [unwired: 6 in, 1 out]
                                }
                                n3101 = local write "Table VRN"(w7264) -> ()
                                n3102 = local write "Table Error"(w7263) -> ()
                                }
                                }
                                }
                                }
                              }
                            }
                          }
                          frame #1 {
                            # "Pas certain que ce soit une\nbonne idée ... devrait être\nenvoyé en même temps <<"
                            n3103 = disable-structure shown="Disabled" {
                              frame Disabled {
                                n3104 = local write "CurvCorrect"(TRUE ("CurvCorrect")) -> ()
                              }
                              frame Enabled {
                              }
                            }
                          }
                        }
                      }
                    }
                  }
                }
              }
              event "enfoncé": Value Change {
                n3105 = event-data() -> ()  [unwired: 1 in, 6 out]
                n3106 = local read "act_cible"() -> (w7282:bool)
                n3107 = local read "act_sonde"() -> (w7281:bool)
                n3108 = Not(x=w7281) -> (.not. x?=w7284:bool)
                n3109 = Not(x=w7282) -> (.not. x?=w7283:bool)
                n3110 = local write "enfoncé"(FALSE ("enfoncé")) -> ()
                n3111 = local write "act_sonde"(w7284) -> ()
                n3112 = local write "act_cible"(w7283) -> ()
              }
              event "Obslib": Mouse Up {
                n3113 = event-data() -> ()  [unwired: 1 in, 7 out]
                n3114 = property on="Librairie des objets" class="Tbl (strict)"() -> ("Selection Start"=w7288:T44, "Selection Size"=w7287:T44)  [unwired: 2 in, 2 out]
                n3115 = Unbundle(w7288) -> ("Row"=w7304:i32)  [unwired: 1 out]
                n3116 = Unbundle(w7287) -> ("Row"=w7303:i32)  [unwired: 1 out]
                n3117 = property on="Obslib" class="Tbl (strict)"() -> ("Selection Start"=w7292:T44, "Selection Size"=w7291:T44)  [unwired: 2 in, 2 out]
                n3118 = Add(x=w7304, y=w7303) -> (x+y=w7302:i32)
                n3119 = Unbundle(w7292) -> ("Row"=w7293:i32)  [unwired: 1 out]
                n3120 = Unbundle(w7291) -> ("Row"=w7294:i32)  [unwired: 1 out]
                n3121 = Add(x=w7293, y=w7294) -> (x+y=w7295:i32)
                n3122 = Bundle(1, 9) -> (w7285:cluster{i32, i32})  [unwired: 1 in]
                n3123 = Bundle(w7302, 0) -> (w7286:cluster{i32, i32})  [unwired: 1 in]
                n3124 = property on="Librairie des objets" class="Tbl (strict)"("Selection Start"=w7286, "Selection Size"=w7285) -> ()  [unwired: 2 in, 2 out]
                n3125 = Bundle(1, 9) -> (w7289:cluster{i32, i32})  [unwired: 1 in]
                n3126 = Bundle(w7295, 0) -> (w7290:cluster{i32, i32})  [unwired: 1 in]
                n3127 = property on="Obslib" class="Tbl (strict)"("Selection Start"=w7290, "Selection Size"=w7289) -> ()  [unwired: 2 in, 2 out]
              }
              event "Reference X": Value Change {
                n3128 = event-data() -> ("OldVal"=w7309:dbl, "NewVal"=w7307:dbl)  [unwired: 1 in, 4 out]
                n3129 = In Range and Coerce(upper limit=725000, x=w7307, lower limit=575000 ("upper limit")) -> (In Range?=w7308:bool)  [unwired: 1 out]
                n3130 = case shown="Faux" w7308 {
                  tunnel: w7309 -> [w7310 _]
                  frame False {
                    n3131 = Two Button Dialog(message="Vous avez mis des valeurs de centres qui semble bizarres,\nVoulez-vous vraiment utiliser celles-ci comme valeurs de centres ?", 1:"NON" ("F button name (\"Cancel\")"), 2:"OUI" ("T button name (\"OK\")")) -> (T button?=w7311:bool)
                    n3132 = case shown="Vrai" w7311 {
                      tunnel: w7310 -> [w7315 _]
                      frame False {
                        n3133 = local write "Reference X"(w7315) -> ()
                      }
                      frame True {
                        n3134 = control-ref of="TERMINAL"() -> (w7316:refnum<vi>)
                        n3135 = control-ref of="Indicateur d'état"() -> (w7317:refnum<vi>)
                        n3136 = call "TERMINAL.vi"("Indicateur Refnum"=w7317, "Terminal Refnum"=w7316, "Indicateur d'état"="Modification des valeurs en X pour le centre instrumental" ("T button name (\"OK\")")) -> ()
                      }
                    }
                  }
                  frame True {
                  }
                }
              }
              event "Reference Y": Value Change {
                n3137 = event-data() -> ("OldVal"=w7323:dbl, "NewVal"=w7321:dbl)  [unwired: 1 in, 4 out]
                n3138 = In Range and Coerce(upper limit=150000 ("lower limit"), x=w7321, lower limit=0 ("upper limit")) -> (In Range?=w7322:bool)  [unwired: 1 out]
                n3139 = case shown="Faux" w7322 {
                  tunnel: w7323 -> [w7324 _]
                  frame False {
                    n3140 = Two Button Dialog(message="Vous avez mis des valeurs de centres qui semble bizarres,\nVoulez-vous vraiment utiliser celles-ci comme valeurs de centres ?", 1:"NON" ("F button name (\"Cancel\")"), 2:"OUI" ("T button name (\"OK\")")) -> (T button?=w7325:bool)
                    n3141 = case shown="Vrai" w7325 {
                      tunnel: w7324 -> [w7329 _]
                      frame False {
                        n3142 = local write "Reference Y"(w7329) -> ()
                      }
                      frame True {
                        n3143 = control-ref of="TERMINAL"() -> (w7330:refnum<vi>)
                        n3144 = control-ref of="Indicateur d'état"() -> (w7331:refnum<vi>)
                        n3145 = call "TERMINAL.vi"("Indicateur Refnum"=w7331, "Terminal Refnum"=w7330, "Indicateur d'état"="Modification des valeurs en Y pour le centre instrumental" ("T button name (\"OK\")")) -> ()
                      }
                    }
                  }
                  frame True {
                  }
                }
              }
              event "load-histo(L)": Mouse Up {
                n3146 = event-data() -> ()  [unwired: 1 in, 8 out]
                n3147 = case shown="Vrai" "load-histo(L)" {
                  frame False {
                  }
                  frame True {
                    n3148 = property on="Librairie des objets" class="Tbl (strict)"() -> ("Selection Start"=w7341:T44)  [unwired: 2 in, 2 out]
                    n3149 = local read "Librairie des objets"() -> (w7339:string[][])
                    n3150 = local write "load-histo(L)"(FALSE ("Charger le l'objet #1")) -> ()
                    n3151 = Unbundle(w7341) -> ("Row"=w7355:i32)  [unwired: 1 out]
                    n3152 = local write "MainTab"(u32 0) -> ()
                    n3153 = Index Array(array=w7339, index (row)=w7355) -> (element=w7338:string[])  [unwired: 1 in]
                    n3154 = Index Array(array=w7338, index #1=2, index #2=3, index #3=4) -> (element #1=w7352:string, element #2=w7353:string, element #3=w7354:string)
                    n3155 = Concatenate Strings("Désirez-vous charger la coordonnées : \nRA = ", w7352, "\nDEC = ", w7353, "\nEpoch = ", w7354) -> (w7347:string)
                    n3156 = Two Button Dialog(message=w7347, 1:"NON" ("F button name (\"Cancel\")"), 2:"OUI" ("T button name (\"OK\")")) -> (T button?=w7351:bool)
                    n3157 = case shown="Vrai" w7351 {
                      tunnel: w7352 -> [_ w7362]
                      tunnel: w7353 -> [_ w7361]
                      tunnel: w7354 -> [_ w7360]
                      tunnel: w7338 -> [_ w7359]
                      tunnel: w7338 -> [_ w7357]
                      frame False {
                      }
                      frame True {
                        n3158 = flat-sequence {
                          tunnel: w7362 -> [w7384]
                          tunnel: w7361 -> [w7383]
                          tunnel: w7360 -> [w7382]
                          tunnel: w7359 -> [w7407]
                          tunnel: [w7398] -> w7358
                          tunnel: w7358 -> [w7414]
                          tunnel: w7357 -> [w7415]
                          frame #0 {
                            w7388 = ", "
                            w7390 = 3600.0 ("y")
                            n3159 = call "time-str-to-time-dbl-RA.vi"("Chaîne"=w7384) -> ("TCS_coords"=w7366:dbl)
                            n3160 = call "time-str-to-time-dbl-DEC.vi"("Chaîne"=w7383) -> ("TCS_coords"=w7364:dbl)
                            n3161 = call "time-str-to-time-dbl.vi"("Chaîne"=w7382) -> ("TCS_coords"=w7371:dbl)
                            n3162 = local read "LST"() -> (w7379:dbl)
                            n3163 = Multiply(x=w7366, y=w7390) -> (x*y=w7381:dbl)
                            n3164 = Multiply(x=w7364, y=w7390) -> (x*y=w7380:dbl)
                            n3165 = control-ref of="TERMINAL"() -> (w7385:refnum<vi>)
                            n3166 = control-ref of="Indicateur d'état"() -> (w7386:refnum<vi>)
                            n3167 = control-ref of="TCS actif"() -> (w7369:refnum<vi>)
                            n3168 = local read "TCS VRN"() -> (w7375:refnum<visa-resource-name>)
                            n3169 = Build Array(w7366, w7364, w7371) -> (w7372:dbl[])
                            n3170 = Format Into String(w7366) -> (resulting string=w7365:string)  [unwired: 3 in, 1 out]
                            n3171 = Format Into String(w7364) -> (resulting string=w7363:string)  [unwired: 3 in, 1 out]
                            n3172 = call "Object_properties.vi"("Target RA"=w7381, "Target DEC"=w7380, "Target Epoch"=w7371, "Sideral Time"=w7379) -> ("NO RA"=w7367:string, "NO DEC"=w7368:string, "NO Epoch"=w7378:dbl, "NO HA"=w7377:dbl, "NO AM"=w7376:dbl)  [unwired: 7 in]
                            n3173 = Concatenate Strings("Chargement de l'objet : ", w7384, w7388, w7383, w7388, w7382) -> (w7389:string)
                            n3174 = call "EXCOM-CMD.vi"("VRN IN"=w7375, "Bool Refnum"=w7369, "Commande #"=6, "Args"=w7372) -> ("VRN OUT"=w7373:refnum<visa-resource-name>, "Error OUT"=w7370:errorcluster)  [unwired: 9 in, 1 out]
                            n3175 = local write "TCS Error"(w7370) -> ()
                            n3176 = local write "Dec_DC"(w7363) -> ()
                            n3177 = local write "AD_DC"(w7365) -> ()
                            n3178 = call "TERMINAL.vi"("Indicateur Refnum"=w7386, "Terminal Refnum"=w7385, "Indicateur d'état"=w7389) -> ()
                            n3179 = local write "TCS VRN"(w7373) -> ()
                            n3180 = local write "NO epoch"(w7378) -> ()
                            n3181 = local write "NO AM"(w7376) -> ()
                            n3182 = local write "NO HA"(w7377) -> ()
                            n3183 = local write "N.O. Déc."(w7368) -> ()
                            n3184 = local write "N.O. A.D."(w7367) -> ()
                          }
                          frame #1 {
                            w7393 = "\\r"
                            n3185 = local read "Numero_DC"() -> (w7396:string)
                            n3186 = local read "Nom_DC"() -> (w7395:string)
                            n3187 = local read "AD_DC"() -> (w7394:string)
                            n3188 = local read "Dec_DC"() -> (w7392:string)
                            n3189 = Index Array(array=w7407, index #1=4 ("index"), index #2=5 ("index")) -> (element #1=w7403:string, element #2=w7404:string)
                            n3190 = Not Equal?(x=w7404, y="") -> (x != y?=w7400:bool)
                            n3191 = Not Equal?(x="", y=w7403) -> (x != y?=w7401:bool)
                            n3192 = local write "From library"(TRUE) -> ()
                            n3193 = Concatenate Strings(w7396, w7393, w7395, w7393, w7394, w7393, w7392) -> (w7391:string)
                            n3194 = Or(x=w7401, y=w7400) -> (x .or. y?=w7399:bool)
                            n3195 = case shown="Vrai" w7399 {
                              selector: w7399 -> [w7409 _]
                              tunnel: [w7409 w7410] -> w7398
                              frame False {
                              }
                              frame True {
                                n3196 = Two Button Dialog(message="Désirez-vous également charger\nles paramètres de guidage ?  ", 1:"NON" ("F button name (\"Cancel\")"), 2:"OUI" ("T button name (\"OK\")")) -> (T button?=w7410:bool)
                              }
                            }
                            n3197 = local write "DC String"(w7391) -> ()
                          }
                          frame #2 {
                            n3198 = case shown="Vrai" w7414 {
                              tunnel: w7415 -> [_ w7427]
                              frame False {
                              }
                              frame True {
                                w7418 = 60.0 ("x")
                                n3199 = call "Time-str-array-to-time-dbl-array.vi"("Array-str"=w7427) -> ("Array-dbl"=w7428:dbl[])
                                n3200 = Index Array(array=w7428, index #1=4, index #2=5, index #3=0 ("index"), index #4=1 ("index"), index #5=6 ("index"), index #6=7 ("index")) -> (element #1=w7432:dbl, element #2=w7430:dbl, element #3=w7431:dbl, element #4=w7429:dbl, element #5=w7424:dbl, element #6=w7423:dbl)
                                n3201 = To Single Precision Float(number=w7424) -> (single precision float=w7421:sgl)
                                n3202 = To Single Precision Float(number=w7423) -> (single precision float=w7422:sgl)
                                n3203 = local write "XReference"(w7421) -> ()
                                n3204 = local write "YReference"(w7422) -> ()
                                n3205 = Subtract(x=w7432, y=w7431) -> (x-y=w7419:dbl)
                                n3206 = Subtract(x=w7430, y=w7429) -> (x-y=w7420:dbl)
                                n3207 = Multiply(x=w7418, y=w7419) -> (x*y=w7416:dbl)
                                n3208 = Multiply(x=w7418, y=w7420) -> (x*y=w7417:dbl)
                                n3209 = property on="TableXYPos" class="GraphXY (strict)"("Cursor.Cursor Position:Cursor X"=w7416, "Cursor.Cursor Position:Cursor Y"=w7417) -> ()  [unwired: 2 in, 2 out]
                              }
                            }
                          }
                        }
                      }
                    }
                    n3210 = Index Array(array=w7338, index #1=0 ("index"), index #2=1 ("index")) -> (element #1=w7334:string, element #2=w7335:string)
                    n3211 = local write "Numero_DC"(w7334) -> ()
                    n3212 = local write "Nom_DC"(w7335) -> ()
                  }
                }
              }
              event "SET ZERO": Mouse Up {
                n3213 = event-data() -> ()  [unwired: 1 in, 8 out]
                n3214 = local read "MC-BonOMM VRN"() -> (w7440:refnum<visa-resource-name>)
                n3215 = call "MC-BonOMM_talker.vi"("MC-BonOMM VRN"=w7440, "Commande"="z" ("write buffer"), "Timeout (ms)"=1000, "answer=command?"=TRUE) -> ("ok ?"=w7437:bool)  [unwired: 1 in, 1 out]
                n3216 = local write "MC_connect"(w7437) -> ()
                n3217 = case shown="Vrai" w7437 {
                  frame False {
                    n3218 = One Button Dialog(message="Erreur lors de la mise à zéro", button name ("OK")="OK ?!?") -> ()  [unwired: 1 out]
                  }
                  frame True {
                  }
                }
              }
              event "ST_RAZ": Mouse Up {
                n3219 = event-data() -> ()  [unwired: 1 in, 8 out]
                n3220 = local read "MC-BonOMM VRN"() -> (w7447:refnum<visa-resource-name>)
                n3221 = call "MC-BonOMM_talker.vi"("MC-BonOMM VRN"=w7447, "Commande"="p" ("write buffer"), "Timeout (ms)"=10000, "answer=command?"=TRUE) -> ("ok ?"=w7444:bool)  [unwired: 1 in, 1 out]
                n3222 = local write "MC_connect"(w7444) -> ()
                n3223 = case shown="Faux" w7444 {
                  frame False {
                    n3224 = One Button Dialog(message="Délai dépasser !?!", button name ("OK")="Heu, ok ?!?") -> ()  [unwired: 1 out]
                  }
                  frame True {
                  }
                }
              }
              event "ST_SPD": Mouse Up {
                n3225 = event-data() -> ()  [unwired: 1 in, 8 out]
                n3226 = local read "MC-BonOMM VRN"() -> (w7452:refnum<visa-resource-name>)
                n3227 = call "Change_speed.vi"("ST_SPD"="ST_SPD", "MC-BonOMM VRN"=w7452) -> ("Connected?"=w7451:bool)
                n3228 = local write "MC_connect"(w7451) -> ()
                n3229 = case shown="Faux" w7451 {
                  frame False {
                    n3230 = property on="Périphérique" class="MDér (strict)"("Value (Signaling)"=u16 3) -> ()  [unwired: 2 in, 2 out]
                  }
                  frame True {
                  }
                }
              }
              event "Load-library": Value Change {
                n3231 = event-data() -> ()  [unwired: 1 in, 6 out]
                n3232 = local write "Load-library"(FALSE ("Load-library")) -> ()
                n3233 = case shown="Vrai" "Load-library" {
                  frame False {
                  }
                  frame True {
                    # "Chemin à confirmer,\nvoir avec Mr Turbide ..."
                    n3234 = local read "path_libdir"() -> (w7458:path)
                    n3235 = File Dialog(6:"*" ("pattern"), 7:"Sélectionner la libraire désirée ..." ("prompt"), 11:w7458) -> (0:w7457:errorcluster, 2:w7462:bool, 3:w7459:path)  [unwired: 4 in, 1 out]
                    n3236 = Unbundle(w7457) -> ()  [unwired: 3 out]
                    n3237 = case shown="Vrai" w7462 {
                      tunnel: w7459 -> [_ w7464]
                      frame False {
                      }
                      frame True {
                        n3238 = local write "Load-library"(FALSE) -> ()
                        n3239 = local write "loaded_lib"(w7464) -> ()
                        n3240 = Strip Path(path=w7464) -> (stripped path=w7467:path)  [unwired: 1 out]
                        n3241 = local read "LST"() -> (w7465:dbl)
                        n3242 = call "Read_obs_files.vi"("Path"=w7464) -> ("Output Table"=w7466:string[][])  [unwired: 1 out]
                        n3243 = for {
                          tunnel: w7466 -> [w7480] mode=indexing
                          tunnel: w7465 -> [w7481]
                          tunnel: [w7477] -> w7463 mode=indexing
                          n3244 = Index Array(array=w7480, index #1=2 ("index"), index #2=3 ("index")) -> (element #1=w7483:string, element #2=w7482:string)
                          n3245 = call "Airmass.vi"("temps sidéral"=w7481, "DEC"=w7482, "RA"=w7483) -> ("airmass"=w7478:dbl)
                          n3246 = Number To Fractional String(number=w7478, precision (6)=i16 2) -> (F-format string=w7479:string)  [unwired: 2 in]
                          n3247 = Insert Into Array(array=w7480, index=5, new element=w7479) -> (w7477:string[])
                        }
                        "Librairie complète" <- w7463
                        "Librairie des objets" <- w7463
                        n3248 = Path To String(path=w7467) -> (string=w7468:string)
